vi "Set Accesss Mode.vi"(10 "Accesss Mode":T1(ring), 11 "Reply Protocol DataSocket in":refnum<class "Reply Protocol DataSocket.lvclass">) -> (3 "Reply Protocol DataSocket out":refnum<class "Reply Protocol DataSocket.lvclass">)   [LabVIEW 2023, in "HAL GOOP4.lvlib" / "Reply Protocol DataSocket.lvclass"]
uses:
  Reply Protocol DataSocket.lvclass
  Reply Protocol DataSocket.lvclass/Reply Protocol DataSocket.ctl
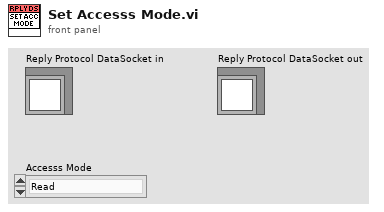
[diagram p1: front panel]
types:
  T1 = enum16{"Read", "Write", "ReadWrite", "BufferedRead", "BufferedReadWrite"}
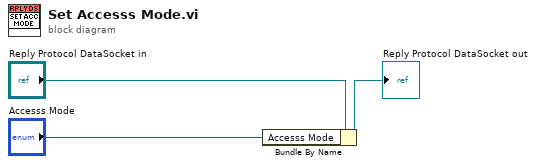
[diagram p0: block diagram]
diagram:
  n1 = Bundle By Name(cluster="Reply Protocol DataSocket in", "Accesss Mode"="Accesss Mode") -> (→"Reply Protocol DataSocket out":refnum<class "Reply Protocol DataSocket.lvclass">)
